vi "Panel.vi"() -> ()   [LabVIEW 2021]
uses:
  Mete.ctl
panel:
  in  "Slide":u32(slide) scale=0.0..8000.0
  in  "stop":bool
  out "Gauge":T1 scale=0.0..8000.0
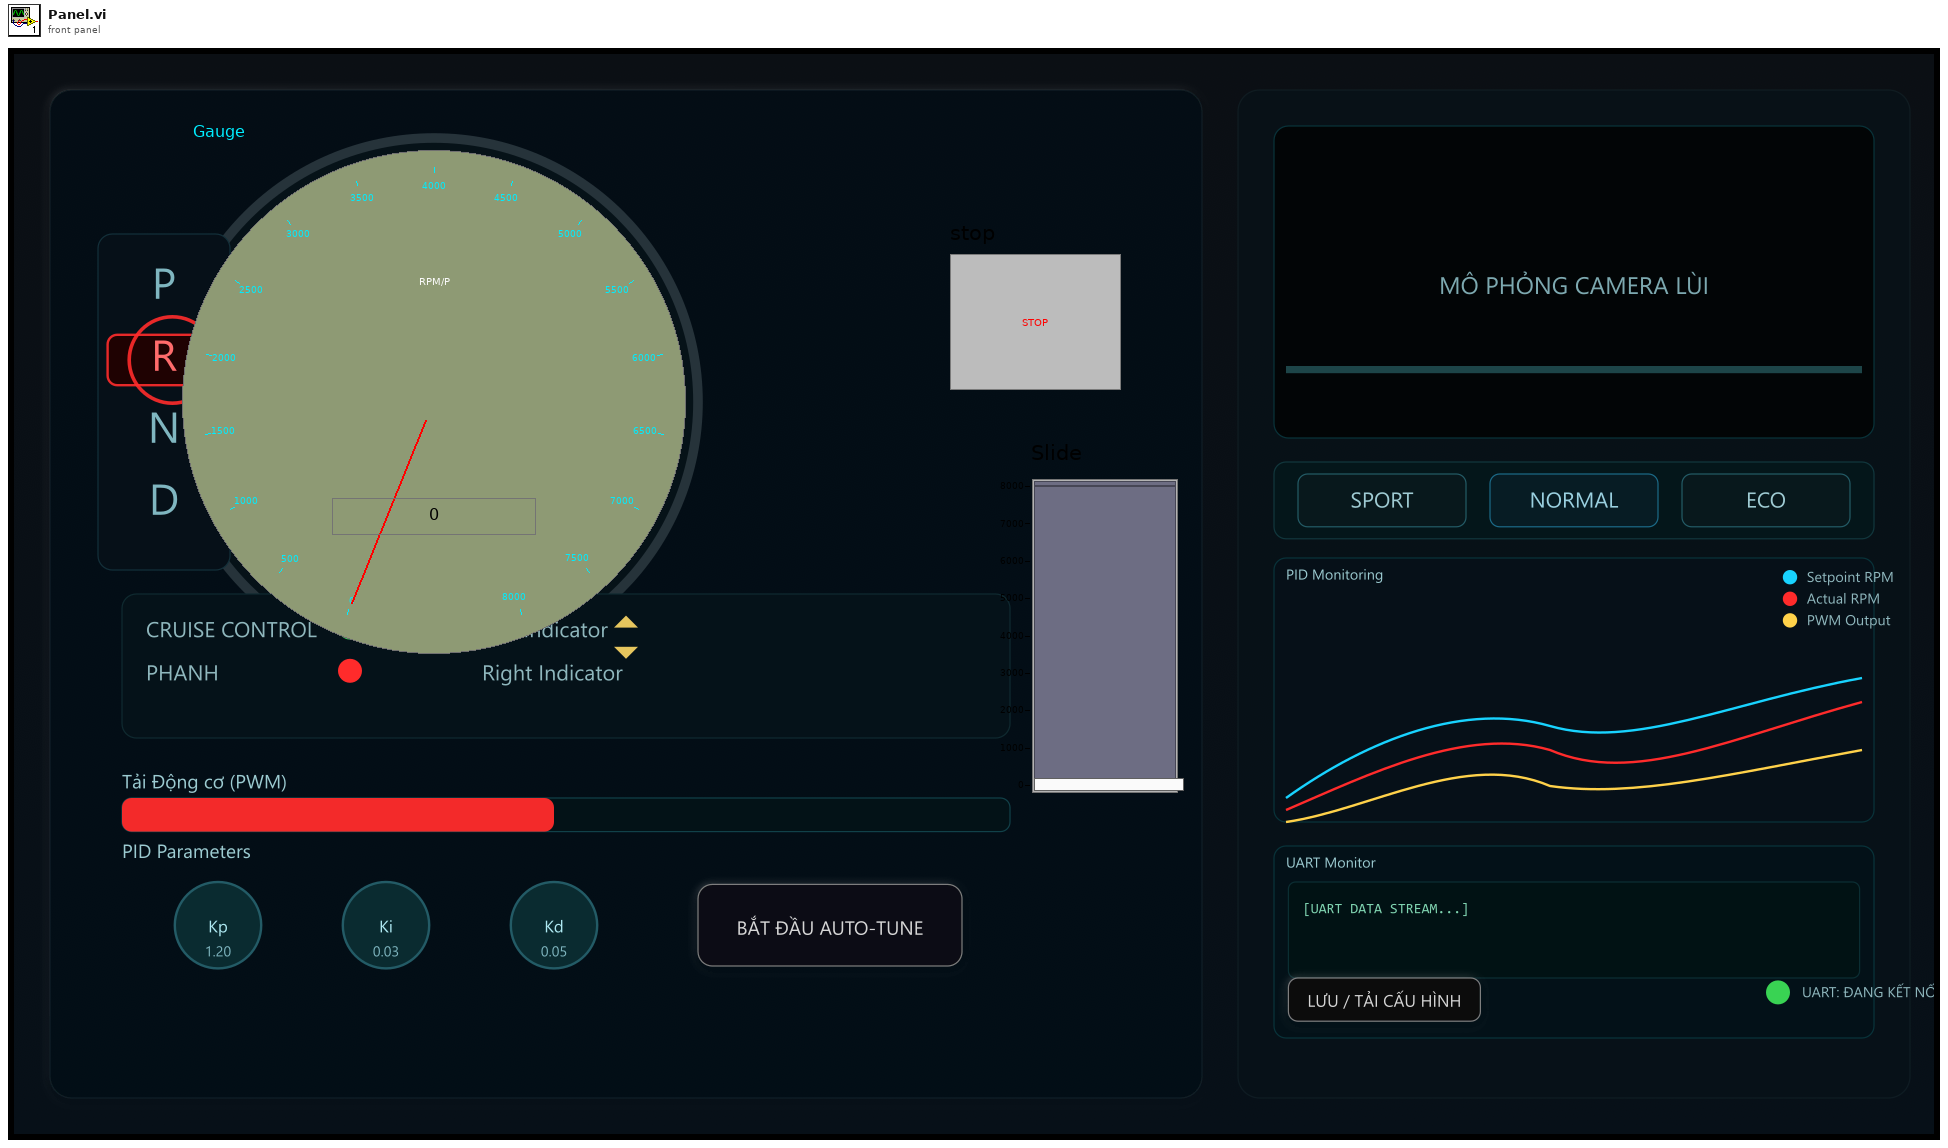
[diagram p1: front panel]
types:
  T1 = typedef "Mete.ctl" = u16
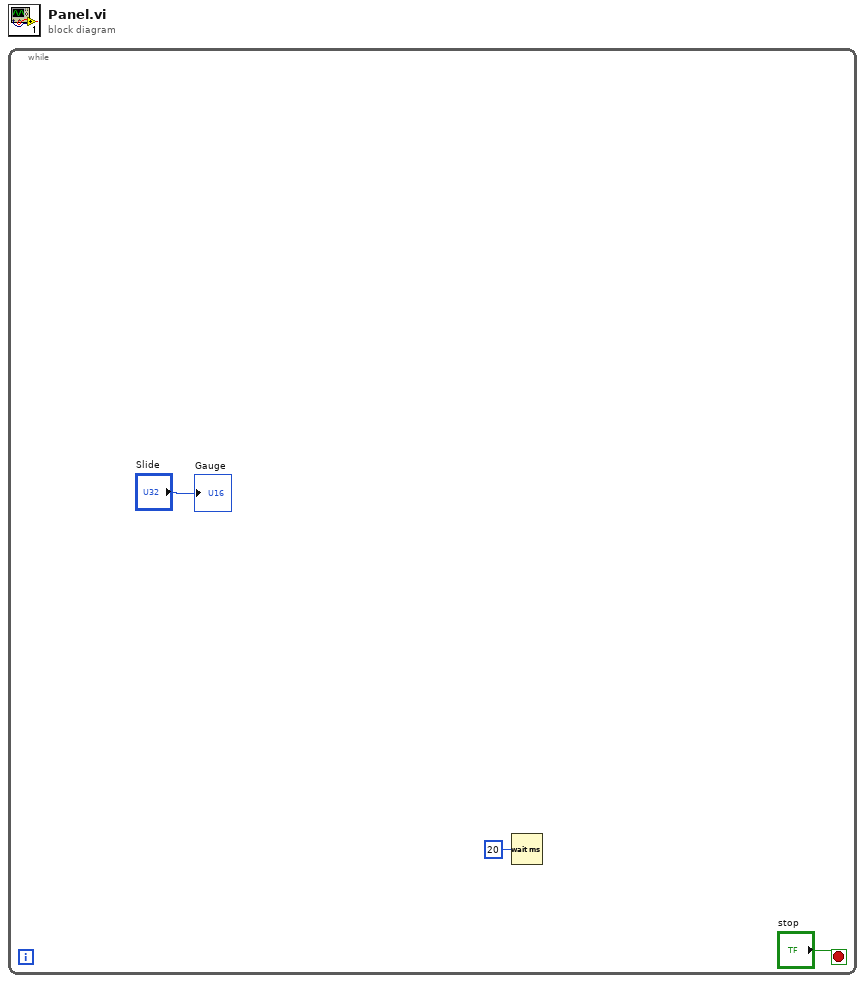
[diagram p0: block diagram]
diagram:
  n1 = while {
    stop <- "stop" stop-if-true
    n2 = Wait (ms)(milliseconds to wait=u32 20) -> ()  [unwired: 1 out]
    "Gauge" <- "Slide"
  }
